vi "test select valid ref.vi"() -> ()   [LabVIEW 2017]
uses:
  446892c7-92f5-466c-bd15-05cfa252f34f.vi
panel:
  out "Non-Empty Number/Path/Refnum":refnum<vi>
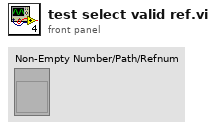
[diagram p1: front panel]
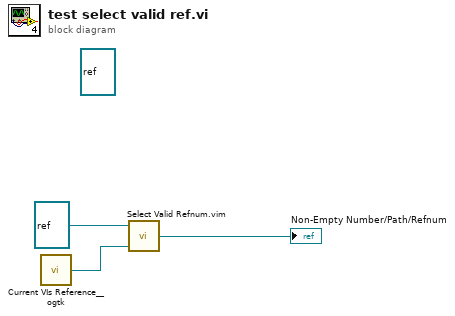
[diagram p0: block diagram]
diagram:
  (unwired) refnum<vi> refnum ("Current VI's reference")
  n1 = call <userlib>:"Current VIs Reference__ogtk.vi"() -> ("Current VI's reference"=w1:refnum<vi>)  [unwired: 5 in]
  n2 = call "Select Valid Refnum.vim"("Referred Number/Path/Refnum"=refnum<vi> refnum ("Current VI's reference"), "Number/Path/Refnum"=w1) -> ("Non-Empty Number/Path/Refnum"=→"Non-Empty Number/Path/Refnum":refnum<vi>)  [unwired: 3 in]
